vi "getLayerDimensions.vi"(0 "error in (no error)":errorcluster, 1 "layer":u32, 2 "ptr":i64) -> (3 "error out":errorcluster, 4 "ptr out":i64, 5 "rows out":u32, 6 "cols out":u32)   [LabVIEW 2016, in "CNet.lvlib"]
uses:
  CNet.lvlib
  Users/jg754/Documents/Visual Studio 2015/Projects/CLearn/x64/Release/CLearn.dll
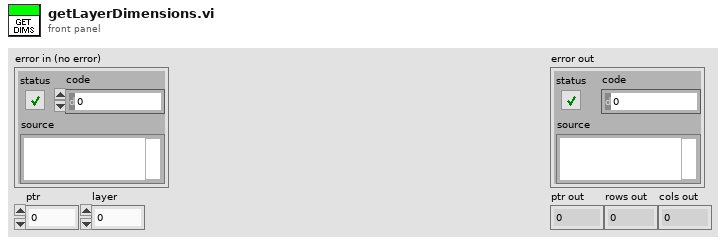
[diagram p1: front panel]
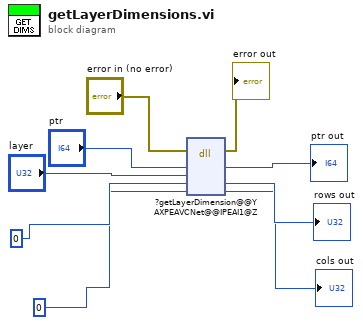
[diagram p0: block diagram]
diagram:
  n1 = dll-call lib="C:/Users/jg754/Documents/Visual Studio 2015/Projects/CLearn/x64/Release/CLearn.dll" fn="?getLayerDimension@@YAXPEAVCNet@@IPEAI1@Z"(error in="error in (no error)", "ptr"="ptr", "layer"="layer", "rows"=u32 0, "cols"=u32 0) -> (error out=→"error out":errorcluster, "ptr"=→"ptr out":i64, "rows"=→"rows out":u32, "cols"=→"cols out":u32)  [unwired: 4 in, 1 out]
